vi "Queue_ReadResponse_Launch.vi"(7 "Queue In [create if empty]":refnum<queue>, 8 "error in (no error)":errorcluster, 11 "HttpResponseMessage in":refnum<class "HttpResponseMessage.lvclass">) -> (0 "error out":errorcluster, 3 "Queue Out":refnum<queue>)   [LabVIEW 2018, in "LabVIEWHTTPClient_NET.lvlib" / "LabVIEWHTTPClient_NET.lvclass"]
uses:
  LabVIEWHTTPClient_NET.lvclass
  HttpResponseMessage/HttpResponseMessage.lvclass
  HttpResponseMessage/Types/ResponseMessage_Cluster.ctl
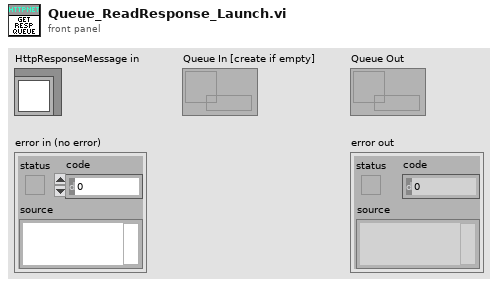
[diagram p1: front panel]
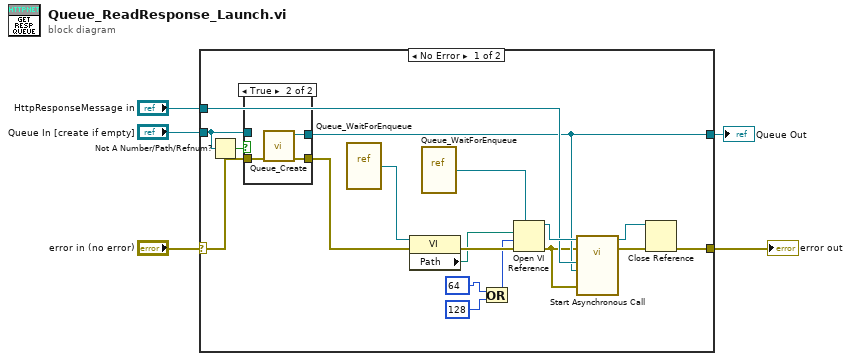
[diagram p0: block diagram]
diagram:
  n1 = case shown="No Error" "error in (no error)" {
    selector: "error in (no error)" -> [w23 w30]
    tunnel: [w7 w30] -> w4
    tunnel: "HttpResponseMessage in" -> [w12 _]
    tunnel: "Queue In [create if empty]" -> [w10 w29]
    tunnel: [w9 w29] -> w1
    frame No Error {
      n2 = Not A Number/Path/Refnum?(number/path/refnum=w10) -> (NaN/Path/Refnum?=w11:bool)
      n3 = case shown="True" w11 {
        tunnel: w23 -> [w24 w28]
        tunnel: [w25 w27] -> w9
        tunnel: [w24 w26] -> w13
        tunnel: w10 -> [w25 _]
        frame False {
        }
        frame True {
          n4 = call "Queue_Create.vi"("error in (no error)"=w28) -> ("error out"=w26:errorcluster, "Queue out"=w27:refnum<queue>)  [unwired: 9 in]
        }
      }
      n5 = vi-ref "Queue_WaitForEnqueue.vi"() -> (w21:refnum<vi>)
      n6 = property class="VI"(reference=w21, error in=w13) -> (error out=w22:errorcluster, "Path"=w20:path)  [unwired: 1 out]
      n7 = vi-ref "Queue_WaitForEnqueue.vi"() -> (w19:refnum<vi>)
      n8 = Or(x=64 ("options"), y=128 ("options")) -> (x .or. y?=w16:i32)
      n9 = Open VI Reference(type specifier VI Refnum (for type only)=w19, vi path=w20, options=w16, error in (no error)=w22) -> (vi reference=w15:refnum<vi>, error out=w8:errorcluster)  [unwired: 2 in]
      n10 = call-by-ref "Start Asynchronous Call"(reference=w15, error in=w8, 8:"error in (no error)"=w8, "Queue in"=w9, "HttpResponseMessage in"=w12) -> (reference out=w6:refnum<vi>, error out=w14:errorcluster)  [unwired: 8 in, 1 out]
      n11 = Close Reference(reference=w6, error in (no error)=w14) -> (error out=w7:errorcluster)
    }
    frame Error {
    }
  }
  "error out" <- w4
  "Queue Out" <- w1
